vi "FlushTcpPort.vi"(6 "max flush time (ms)":i32=5000, 7 "file":bool, 8 "error in (no error)":errorcluster, 11 "connection ID in":T1) -> (0 "error out":errorcluster, 1 "timed out":bool, 2 "data flushed":bool, 3 "connection ID out":T1)   [LabVIEW 2017]
uses:
  <vilib>/addons/InsightCM/MessageBus/TcpApi/controls/TcpMessageReference.ctl
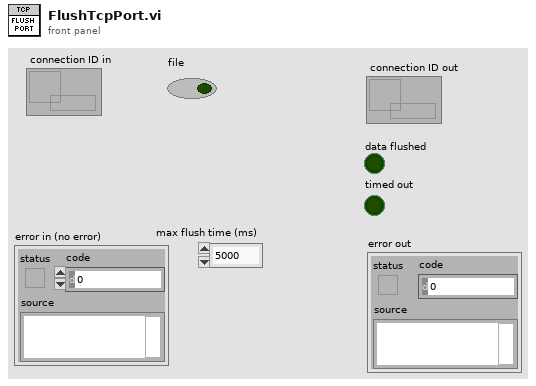
[diagram p1: front panel]
types:
  T1 = typedef "TcpMessageReference.ctl" = refnum<data-value>
  T2 = cluster{"DeviceId":string, "CmdStream":refnum<k5>, "FileStream":refnum<k5>}
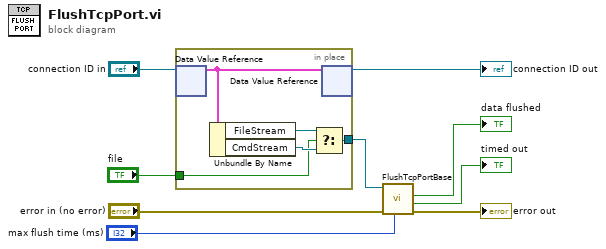
[diagram p0: block diagram]
diagram:
  n1 = in-place {
    in-place-border: "file" -> [w11]
    in-place-border: [w10] -> w5
    n2 = in-place-dvr #1("connection ID in") -> (w14:T2)  [unwired: 1 out]
    n3 = Unbundle By Name(w14) -> ("FileStream"=w13:refnum<k5>, "CmdStream"=w12:refnum<k5>)
    n4 = Select(t=w13, s=w11, f=w12) -> (s? t:f=w10:refnum<k5>)
    n5 = in-place-dvr #1(w14) -> (→"connection ID out":T1)  [unwired: 1 out]
  }
  n6 = call <vilib>:"FlushTcpPortBase.vi"("max flush time (ms)"="max flush time (ms)", "error in (no error)"="error in (no error)", "tcp in"=w5) -> ("error out"=→"error out":errorcluster, "timed out"=→"timed out":bool, "data flushed"=→"data flushed":bool)  [unwired: 5 in, 1 out]
